vi "SailRudderControlLogic.vi"(0 "Robot Heading":dbl, 1 "RelativeWindAngle":dbl, 7 "Waypoint":T3 {"North" format="%#_10f"; "East" format="%#_8f"}, 9 "Robot Location":T3 {"North" format="%#_10f"; "East" format="%#_8f"}, 11 "Commanded Boat Regime":T4) -> (4 "Suggested Sail Setpoints":T2 {"MainSailSuggestion" min=0.0 max=1.0; "JibSailSuggestion" min=0.0 max=1.0}, 15 "Suggested Rudder Setpoint":T1 min=-1.0 max=1.0)   [LabVIEW 2013]
doc: "Spring 2014\n\nGiven the current regime of the boat, the relative wind angle, the wind sped, and the \"desired proportion of boat speed,\" returns the corresponding sail orientation.\n\nGiven the current regime, the waypoint, the boat location, and the boat heading, returns the corresponding rudder orientation."
uses:
  Data/TypeDefs/Boat Regimes.ctl
  Data/TypeDefs/Sailing Regimes.ctl
  Data/TypeDefs/Emergency Regimes.ctl
  Data/TypeDefs/UTM Location.ctl
  Data/TypeDefs/Sail Set Suggestions.ctl
  Data/TypeDefs/Rudder Set Suggestions.ctl
panel:
  in  "Current Main Position":dbl
  in  "DesiredHeading":dbl
  in  "AbsoluteWindAngle":dbl
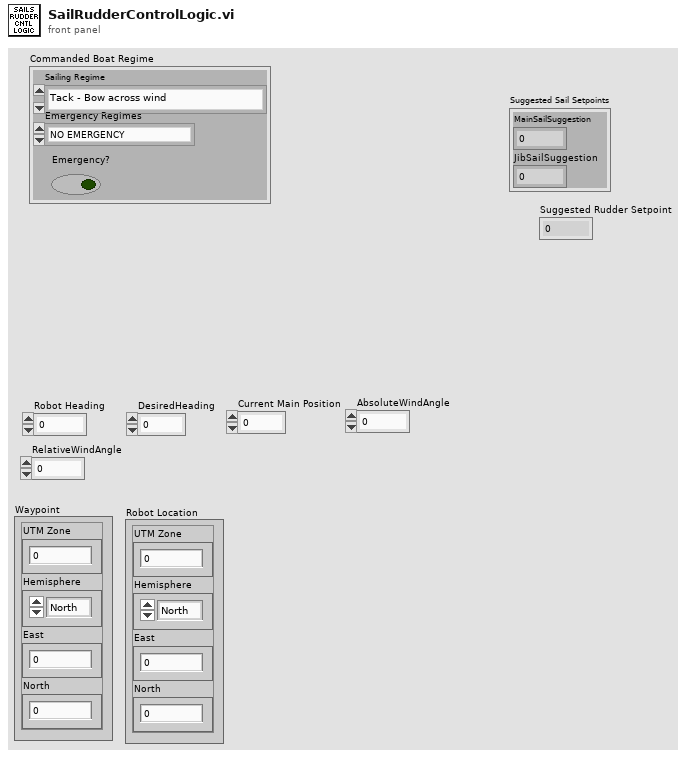
[diagram p1: front panel]
types:
  T1 = typedef "Rudder Set Suggestions.ctl" = dbl
  T2 = typedef "Sail Set Suggestions.ctl" = cluster{"MainSailSuggestion":dbl, "JibSailSuggestion":dbl}
  T3 = typedef "UTM Location.ctl" = cluster{"UTM Zone":dbl, "Hemisphere":enum16{"North", "South"}, "East":dbl, "North":dbl}
  T4 = typedef "Boat Regimes.ctl" = cluster{"Sailing Regime":T5, "Emergency Regimes":T6, "Emergency?":bool}
  T5 = typedef "Sailing Regimes.ctl" = enum16{"Tack - Bow across wind", "Upwind - Starboard Tack", "Turn between Upwind/Reach - Starboard Tack", "Reach - Starboard Tack", "Turn between Reach/Run - Starboard Tack", "Run - Starboard Tack", "Jibe - Stern across wind", "Run - Port Tack", "Turn between Reach/Run - Port Tack", "Reach - Port Tack", "Turn between Upwind/Reach - Port Tack", "Upwind - Port Tack"}
  T6 = typedef "Emergency Regimes.ctl" = enum16{"NO EMERGENCY", "No Knockdown", "Obstacle Avoid"}
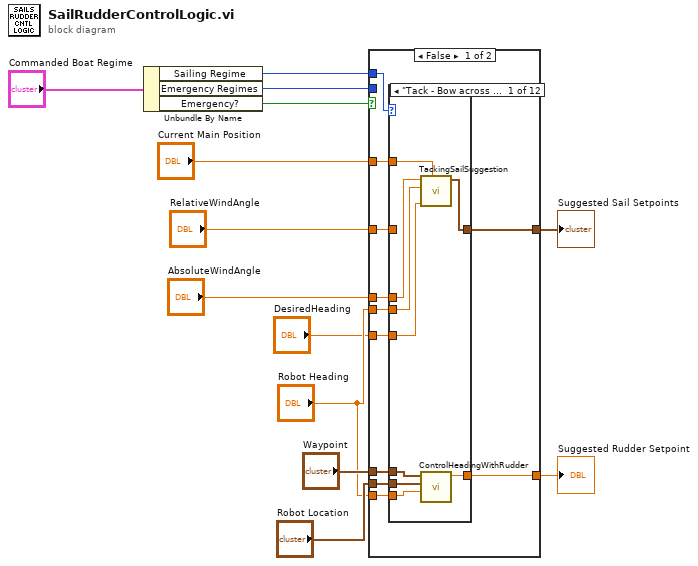
[diagram p0: block diagram]
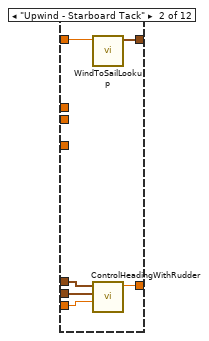
[diagram p2: hidden frame]
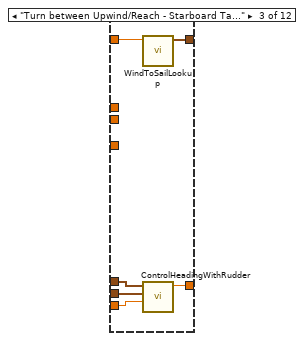
[diagram p3: hidden frame]
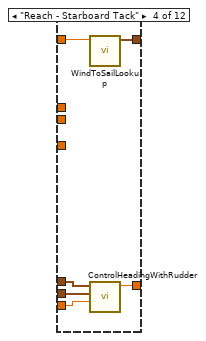
[diagram p4: hidden frame]
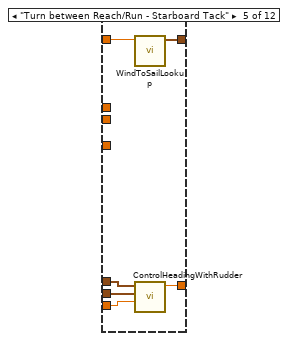
[diagram p5: hidden frame]
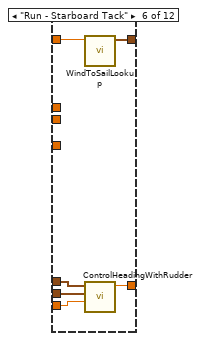
[diagram p6: hidden frame]
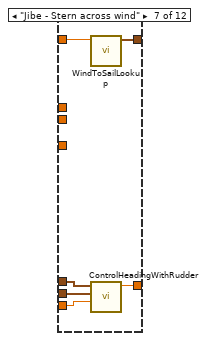
[diagram p7: hidden frame]
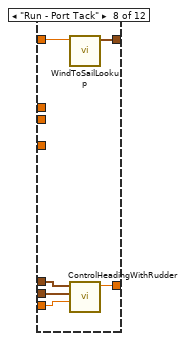
[diagram p8: hidden frame]
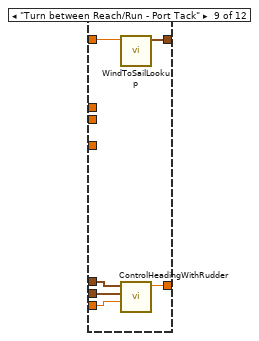
[diagram p9: hidden frame]
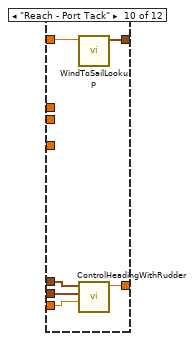
[diagram p10: hidden frame]
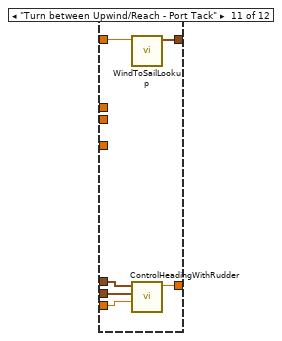
[diagram p11: hidden frame]
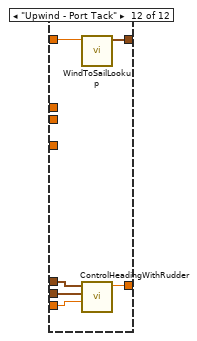
[diagram p12: hidden frame]
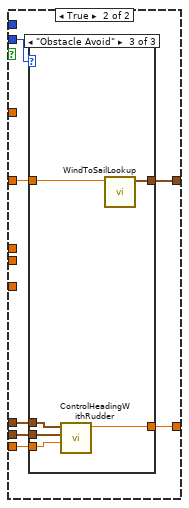
[diagram p13: hidden frame]
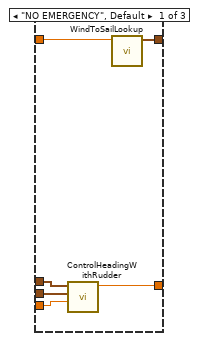
[diagram p14: hidden frame]
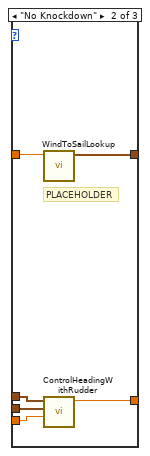
[diagram p15: hidden frame]
diagram:
  n1 = Unbundle By Name("Commanded Boat Regime") -> ("Sailing Regime"=w12:T5, "Emergency Regimes"=w7:T6, "Emergency?"=w13:bool)
  n2 = case shown="False" w13 {
    tunnel: w12 -> [w24 _]
    tunnel: "Waypoint" -> [w23 w103]
    tunnel: "Robot Location" -> [w22 w102]
    tunnel: "Robot Heading" -> [w21 w101]
    tunnel: "RelativeWindAngle" -> [w20 w105]
    tunnel: [w19 w104] -> w6
    tunnel: [w18 w100] -> w5
    tunnel: w7 -> [_ w106]
    tunnel: "Robot Heading" -> [w17 _]
    tunnel: "AbsoluteWindAngle" -> [w16 _]
    tunnel: "DesiredHeading" -> [w15 _]
    tunnel: "Current Main Position" -> [w14 _]
    frame False {
      n3 = case shown="\"Tack - Bow across wind\", Default" w24 {
        tunnel: w23 -> [w33 w39 w44 w50 w56 w61 w67 w75 w79 w87 w91 w99]
        tunnel: w22 -> [w32 w38 w43 w49 w55 w60 w66 w74 w78 w86 w90 w98]
        tunnel: w21 -> [w31 w37 w42 w48 w54 w59 w65 w73 w77 w85 w89 w97]
        tunnel: w20 -> [_ w36 w45 w51 w57 w63 w69 w71 w81 w83 w93 w95]
        tunnel: [w29 w35 w41 w47 w53 w62 w68 w70 w80 w82 w92 w94] -> w19
        tunnel: [w30 w34 w40 w46 w52 w58 w64 w72 w76 w84 w88 w96] -> w18
        tunnel: w17 -> [w28 _ _ _ _ _ _ _ _ _ _ _]
        tunnel: w16 -> [w27 _ _ _ _ _ _ _ _ _ _ _]
        tunnel: w15 -> [w26 _ _ _ _ _ _ _ _ _ _ _]
        tunnel: w14 -> [w25 _ _ _ _ _ _ _ _ _ _ _]
        frame "Tack - Bow across wind", Default {
          n4 = call "TackingSailSuggestion.vi"("Current Main Position"=w25, "DesiredHeading"=w26, "RobotHeading"=w28, "AbsoluteWindAngle"=w27) -> ("Suggested Sail Setpoints"=w29:T2)  [unwired: 7 in]
          n5 = call "ControlHeadingWithRudder.vi"("Waypoint"=w33, "Robot Location"=w32, "Robot Heading"=w31) -> ("Suggested Rudder Setpoint"=w30:T1)  [unwired: 7 in]
        }
        frame "Upwind - Starboard Tack" {
          n6 = call "WindToSailLookup.vi"("RelativeWindAngle"=w36) -> ("Suggested Sail Setpoints"=w35:T2)  [unwired: 10 in]
          n7 = call "ControlHeadingWithRudder.vi"("Waypoint"=w39, "Robot Location"=w38, "Robot Heading"=w37) -> ("Suggested Rudder Setpoint"=w34:T1)  [unwired: 7 in]
        }
        frame "Turn between Upwind/Reach - Starboard Tack" {
          n8 = call "WindToSailLookup.vi"("RelativeWindAngle"=w45) -> ("Suggested Sail Setpoints"=w41:T2)  [unwired: 10 in]
          n9 = call "ControlHeadingWithRudder.vi"("Waypoint"=w44, "Robot Location"=w43, "Robot Heading"=w42) -> ("Suggested Rudder Setpoint"=w40:T1)  [unwired: 7 in]
        }
        frame "Reach - Starboard Tack" {
          n10 = call "WindToSailLookup.vi"("RelativeWindAngle"=w51) -> ("Suggested Sail Setpoints"=w47:T2)  [unwired: 10 in]
          n11 = call "ControlHeadingWithRudder.vi"("Waypoint"=w50, "Robot Location"=w49, "Robot Heading"=w48) -> ("Suggested Rudder Setpoint"=w46:T1)  [unwired: 7 in]
        }
        frame "Turn between Reach/Run - Starboard Tack" {
          n12 = call "WindToSailLookup.vi"("RelativeWindAngle"=w57) -> ("Suggested Sail Setpoints"=w53:T2)  [unwired: 10 in]
          n13 = call "ControlHeadingWithRudder.vi"("Waypoint"=w56, "Robot Location"=w55, "Robot Heading"=w54) -> ("Suggested Rudder Setpoint"=w52:T1)  [unwired: 7 in]
        }
        frame "Run - Starboard Tack" {
          n14 = call "WindToSailLookup.vi"("RelativeWindAngle"=w63) -> ("Suggested Sail Setpoints"=w62:T2)  [unwired: 10 in]
          n15 = call "ControlHeadingWithRudder.vi"("Waypoint"=w61, "Robot Location"=w60, "Robot Heading"=w59) -> ("Suggested Rudder Setpoint"=w58:T1)  [unwired: 7 in]
        }
        frame "Jibe - Stern across wind" {
          n16 = call "WindToSailLookup.vi"("RelativeWindAngle"=w69) -> ("Suggested Sail Setpoints"=w68:T2)  [unwired: 10 in]
          n17 = call "ControlHeadingWithRudder.vi"("Waypoint"=w67, "Robot Location"=w66, "Robot Heading"=w65) -> ("Suggested Rudder Setpoint"=w64:T1)  [unwired: 7 in]
        }
        frame "Run - Port Tack" {
          n18 = call "WindToSailLookup.vi"("RelativeWindAngle"=w71) -> ("Suggested Sail Setpoints"=w70:T2)  [unwired: 10 in]
          n19 = call "ControlHeadingWithRudder.vi"("Waypoint"=w75, "Robot Location"=w74, "Robot Heading"=w73) -> ("Suggested Rudder Setpoint"=w72:T1)  [unwired: 7 in]
        }
        frame "Turn between Reach/Run - Port Tack" {
          n20 = call "WindToSailLookup.vi"("RelativeWindAngle"=w81) -> ("Suggested Sail Setpoints"=w80:T2)  [unwired: 10 in]
          n21 = call "ControlHeadingWithRudder.vi"("Waypoint"=w79, "Robot Location"=w78, "Robot Heading"=w77) -> ("Suggested Rudder Setpoint"=w76:T1)  [unwired: 7 in]
        }
        frame "Reach - Port Tack" {
          n22 = call "WindToSailLookup.vi"("RelativeWindAngle"=w83) -> ("Suggested Sail Setpoints"=w82:T2)  [unwired: 10 in]
          n23 = call "ControlHeadingWithRudder.vi"("Waypoint"=w87, "Robot Location"=w86, "Robot Heading"=w85) -> ("Suggested Rudder Setpoint"=w84:T1)  [unwired: 7 in]
        }
        frame "Turn between Upwind/Reach - Port Tack" {
          n24 = call "WindToSailLookup.vi"("RelativeWindAngle"=w93) -> ("Suggested Sail Setpoints"=w92:T2)  [unwired: 10 in]
          n25 = call "ControlHeadingWithRudder.vi"("Waypoint"=w91, "Robot Location"=w90, "Robot Heading"=w89) -> ("Suggested Rudder Setpoint"=w88:T1)  [unwired: 7 in]
        }
        frame "Upwind - Port Tack" {
          n26 = call "WindToSailLookup.vi"("RelativeWindAngle"=w95) -> ("Suggested Sail Setpoints"=w94:T2)  [unwired: 10 in]
          n27 = call "ControlHeadingWithRudder.vi"("Waypoint"=w99, "Robot Location"=w98, "Robot Heading"=w97) -> ("Suggested Rudder Setpoint"=w96:T1)  [unwired: 7 in]
        }
      }
    }
    frame True {
      n28 = case shown="\"Obstacle Avoid\"" w106 {
        tunnel: w105 -> [w112 w118 w119]
        tunnel: [w107 w117 w120] -> w104
        tunnel: w103 -> [w111 w116 w124]
        tunnel: w102 -> [w110 w115 w123]
        tunnel: w101 -> [w109 w114 w122]
        tunnel: [w108 w113 w121] -> w100
        frame "NO EMERGENCY", Default {
          n29 = call "ControlHeadingWithRudder.vi"("Waypoint"=w111, "Robot Location"=w110, "Robot Heading"=w109) -> ("Suggested Rudder Setpoint"=w108:T1)  [unwired: 7 in]
          n30 = call "WindToSailLookup.vi"("RelativeWindAngle"=w112) -> ("Suggested Sail Setpoints"=w107:T2)  [unwired: 10 in]
        }
        frame "No Knockdown" {
          # "PLACEHOLDER"
          n31 = call "WindToSailLookup.vi"("RelativeWindAngle"=w118) -> ("Suggested Sail Setpoints"=w117:T2)  [unwired: 10 in]
          n32 = call "ControlHeadingWithRudder.vi"("Waypoint"=w116, "Robot Location"=w115, "Robot Heading"=w114) -> ("Suggested Rudder Setpoint"=w113:T1)  [unwired: 7 in]
        }
        frame "Obstacle Avoid" {
          n33 = call "ControlHeadingWithRudder.vi"("Waypoint"=w124, "Robot Location"=w123, "Robot Heading"=w122) -> ("Suggested Rudder Setpoint"=w121:T1)  [unwired: 7 in]
          n34 = call "WindToSailLookup.vi"("RelativeWindAngle"=w119) -> ("Suggested Sail Setpoints"=w120:T2)  [unwired: 10 in]
        }
      }
    }
  }
  "Suggested Sail Setpoints" <- w6
  "Suggested Rudder Setpoint" <- w5
